vi "CmdExe.Generate Measurement based on Exe Return Code.vi"(5 "StdOut is Fail Code":bool, 6 "BaseCode":i32=7000, 7 "Name":string, 8 "Error":errorcluster, 9 "RtnCode":i32, 10 "StdErr":string, 11 "StdOut":string) -> (0 "Success":bool, 3 "Meas":T1 {"Status" items=["LOG", "PASS", "FAIL", "ERROR"]})   [LabVIEW 2024]
uses:
  Results/Result.Measurement Item.ctl
  Results/Result.Measurement and Attribute Item Status.ctl
  Errors/Error.Error Code List.ctl
  Errors.lvlib
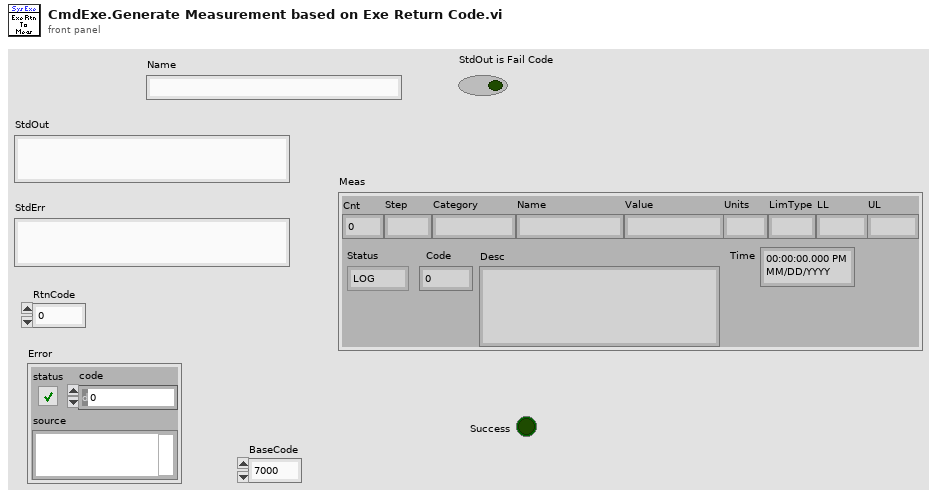
[diagram p1: front panel]
types:
  T1 = typedef "Result.Measurement Item.ctl" = cluster{"Cnt":i32, "Step":string, "Category":string, "Name":string, "Value":string, "Units":string, "LimType":string, "LL":string, "UL":string, "Status":T2, "Code":i32, "Desc":string, "Time":timestamp}
  T2 = typedef "Result.Measurement and Attribute Item Status.ctl" = i32
  T3 = typedef "EQMF.lvlib/Errors.lvlib/Error.Error Code List.ctl" = i32
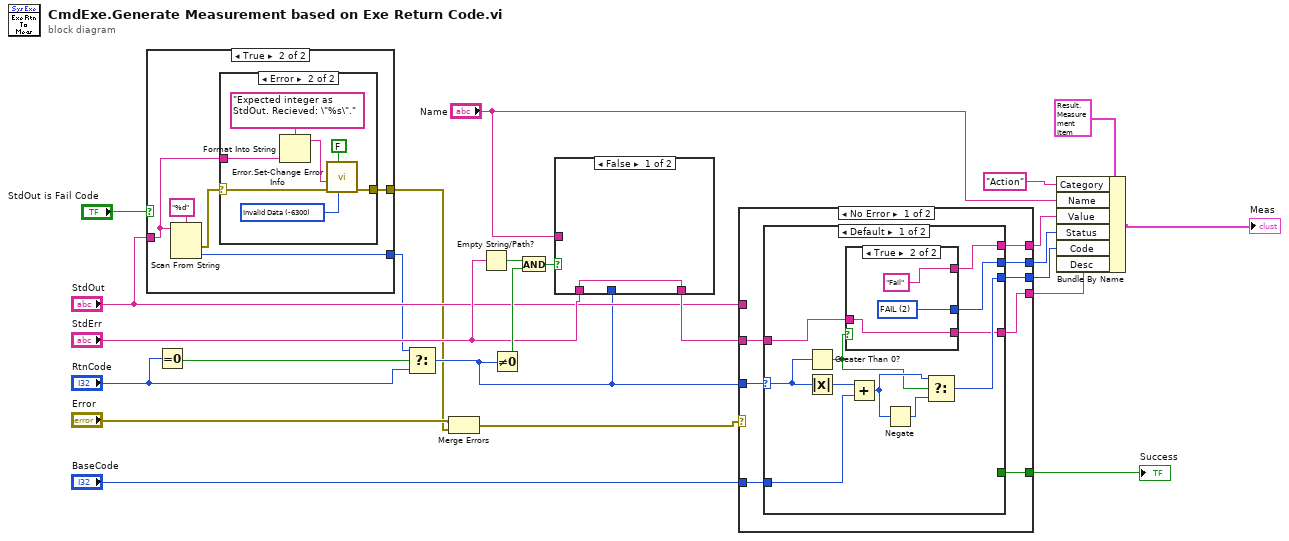
[diagram p0: block diagram]
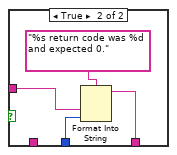
[diagram p4: hidden frame]
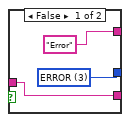
[diagram p5: hidden frame]
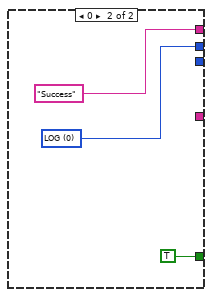
[diagram p6: hidden frame]
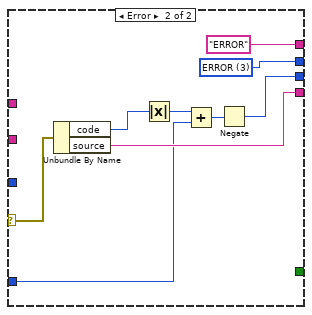
[diagram p7: hidden frame]
diagram:
  n1 = case shown="True" "StdOut is Fail Code" {
    tunnel: "StdOut" -> [_ w25]
    tunnel: [_ w29] -> w7
    tunnel: [_ w26] -> w2
    frame False {
    }
    frame True {
      n2 = Scan From String(format string="%d", input string=w25) -> (error out=w27:errorcluster, output 1=w29:i32)  [unwired: 3 in, 2 out]
      n3 = case shown="Error" w27 {
        selector: w27 -> [_ w36]
        tunnel: [_ w35] -> w26
        tunnel: w25 -> [_ w31]
        frame No Error {
        }
        frame Error {
          w34 = T3 -6300 items=["No Error"=0, "Abort"=-2, "Misc"=-5000, "Fixture Error"=-5100, "File IO - General"=-5200, "FIle IO - Config Error"=-5201, "Instrument - General"=-5300, "Instrument - Serial Com"=-5301, "Instrument - Camera"=-5302, "Instrument - PS"=-5303, "Instrument - Oscilloscope"=-5304, "Instrument - Function Gen"=-5305, "Instrument - Load"=-5306, "Instrument - Meter"=-5307, "Instrument - Power Control"=-5308, "Instrument - Motion"=-5309, "Instrument - RF"=-5310, "System Exe"=-5400, "Image Processing"=-5500, "Communication"=-5600, "Script - Syntax Error"=-6000, "Script - Invalid Name or Param"=-6100, "Script - Timeout"=-6200, "Invalid Data"=-6300, "FW Update Error"=-6500] ("Std Code")
          n4 = Format Into String(format string="Expected integer as StdOut. Recieved: \"%s\".", w31) -> (resulting string=w33:string)  [unwired: 2 in, 1 out]
          n5 = call "Error.Set-Change Error Info.vi"("Std Code"=w34, "Append Details"=FALSE, "error in"=w36, "Description"=w33) -> ("error out"=w35:errorcluster)  [unwired: 7 in]
        }
      }
    }
  }
  n6 = Equal To 0?(x="RtnCode") -> (x = 0?=w6:bool)
  n7 = Select(t=w7, s=w6, f="RtnCode") -> (s? t:f=w4:i32)
  n8 = Merge Errors("Error", w2) -> (w1:errorcluster)
  n9 = Empty String/Path?(string/path="StdErr") -> (empty?=w15:bool)
  n10 = Not Equal To 0?(x=w4) -> (x != 0?=w14:bool)
  n11 = And(x=w15, y=w14) -> (x .and. y?=w12:bool)
  n12 = case shown="False" w12 {
    tunnel: "StdErr" -> [w37 _]
    tunnel: [w37 w40] -> w11
    tunnel: w4 -> [_ w39]
    tunnel: "Name" -> [_ w38]
    frame False {
    }
    frame True {
      n13 = Format Into String(format string="%s return code was %d and expected 0.", w38, w39) -> (resulting string=w40:string)  [unwired: 2 in, 1 out]
    }
  }
  n14 = case shown="No Error" w1 {
    selector: w1 -> [_ w77]
    tunnel: [w48 "ERROR"] -> w22
    tunnel: [w49 w75] -> w19
    tunnel: [w44 w70] -> w21
    tunnel: [w42 w76] -> w20
    tunnel: "BaseCode" -> [w45 w72]
    tunnel: "StdOut" -> [_ _]
    tunnel: w11 -> [w46 _]
    tunnel: w4 -> [w47 _]
    tunnel: [w43 _] -> w16
    frame No Error {
      n15 = case shown="Default" w47 {
        selector: w47 -> [w58 _]
        tunnel: [w51 w69] -> w49
        tunnel: [w52 "Success"] -> w48
        tunnel: w46 -> [w53 _]
        tunnel: w45 -> [w59 _]
        tunnel: [w55 _] -> w44
        tunnel: [_ TRUE] -> w43
        tunnel: [w50 _] -> w42
        frame Default {
          n16 = Greater Than 0?(x=w58) -> (x > 0?=w54:bool)
          n17 = Absolute Value(x=w58) -> (abs(x)=w60:i32)
          n18 = case shown="True" w54 {
            tunnel: w53 -> [w61 w64]
            tunnel: ["Error" "Fail"] -> w52
            tunnel: [w62 w65] -> w51
            tunnel: [w61 w64] -> w50
            frame False {
              w62 = T2 3 items=["LOG", "PASS", "FAIL", "ERROR"] ("Status")
            }
            frame True {
              w65 = T2 2 items=["LOG", "PASS", "FAIL", "ERROR"] ("Status")
            }
          }
          n19 = Add(x=w60, y=w59) -> (x+y=w56:i32)
          n20 = Negate(x=w56) -> (-x=w57:i32)
          n21 = Select(t=w56, s=w54, f=w57) -> (s? t:f=w55:i32)
        }
        frame 0 {
          w69 = T2 0 items=["LOG", "PASS", "FAIL", "ERROR"] ("Status")
        }
      }
    }
    frame Error {
      w75 = T2 3 items=["LOG", "PASS", "FAIL", "ERROR"] ("Status")
      n22 = Unbundle By Name(w77) -> ("code"=w74:i32, "source"=w76:string)
      n23 = Absolute Value(x=w74) -> (abs(x)=w73:i32)
      n24 = Add(x=w73, y=w72) -> (x+y=w71:i32)
      n25 = Negate(x=w71) -> (-x=w70:i32)
    }
  }
  "Success" <- w16
  n26 = Bundle By Name(cluster=T1 {"Cnt"=0, "Step"="", "Category"="", "Name"="", "Value"="", "Units"="", "LimType"="", "LL"="", "UL"="", "Status"=0, "Code"=0, "Desc"="", "Time"=timestamp(0 s since 1904-01-01)} ("Meas"), "Category"="Action", "Name"="Name", "Value"=w22, "Status"=w19, "Code"=w21, "Desc"=w20) -> (→"Meas":T1)
